vi "ifr2025 VOR  (not On Ifr2025).vi"(8 "error in (no error)":errorcluster {"code" format="%.0x"}, 11 "instrument handle":refnum<visa-resource-name>) -> (0 "error out":errorcluster {"code" format="%.0x"}, 1 "REF Depth":dbl, 2 "VOR Depth":dbl, 3 "instrument handle out":refnum<visa-resource-name>, 4 "VORID Depth":dbl, 5 "Direction":i16, 6 "Bearing":dbl)   [LabVIEW 2009]
doc: "Retrieve the current settings for VOR mode."
uses:
  Ifr2025_32.dll
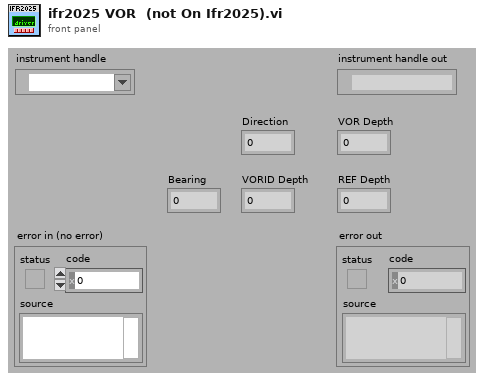
[diagram p1: front panel]
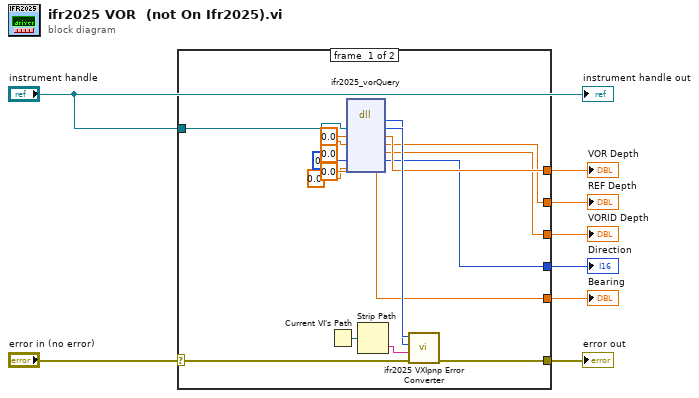
[diagram p0: block diagram]
diagram:
  n1 = case shown="No Error" "error in (no error)" {
    selector: "error in (no error)" -> [w20 w26]
    tunnel: [w19 w26] -> w8
    tunnel: "instrument handle" -> [w24 _]
    tunnel: [w17 _] -> w5
    tunnel: [w15 _] -> w4
    tunnel: [w13 _] -> w3
    tunnel: [w11 _] -> w2
    tunnel: [w9 _] -> w1
    frame #0 {
      n2 = Current VI's Path() -> (path=w25:path)
      n3 = dll-call lib="P:/inst/Marconi 2024 Signal Generator/source/labview/ifr2025/ifr2025/ifr2025_*.*" fn="ifr2025_vorQuery"("vi"=w24, "VOR Depth"=0.0, "REF Depth"=0.0, "VORID Depth"=0.0, "Direction"=i16 0, "Bearing"=0.0) -> (w22:i32, "vi"=w23:u32, "VOR Depth"=w17:dbl, "REF Depth"=w15:dbl, "VORID Depth"=w13:dbl, "Direction"=w11:i16, "Bearing"=w9:dbl)  [unwired: 3 in, 2 out]
      n4 = Strip Path(path=w25) -> (name=w21:string)  [unwired: 1 out]
      n5 = call "ifr2025 VXIpnp Error Converter.vi"("error in (no error)"=w20, "name of VI (\"\")"=w21, "CVI error code (0)"=w22, "instrument handle"=w23) -> ("error out"=w19:errorcluster)  [unwired: 7 out]
    }
    frame #1 {
    }
  }
  "error out" <- w8
  "VOR Depth" <- w5
  "REF Depth" <- w4
  "VORID Depth" <- w3
  "Direction" <- w2
  "Bearing" <- w1
  "instrument handle out" <- "instrument handle"
